vi "Oven_Con_Status.vi"() -> ()   [LabVIEW 2017]
uses:
  99af3ae5-4f0b-4404-ba7d-ed1d743938f4.vi
  <vilib>/addons/database/Connection.llb/DB Tools Open Connec (Path).vi
  <vilib>/addons/database/NI_Database_API.lvlib
panel:
  out "subarray":string[](array[string])
  out "index of element":i32
  out "output array":string[](array[string])
  out "data":string[][](array[string])
  out "error out 4":errorcluster
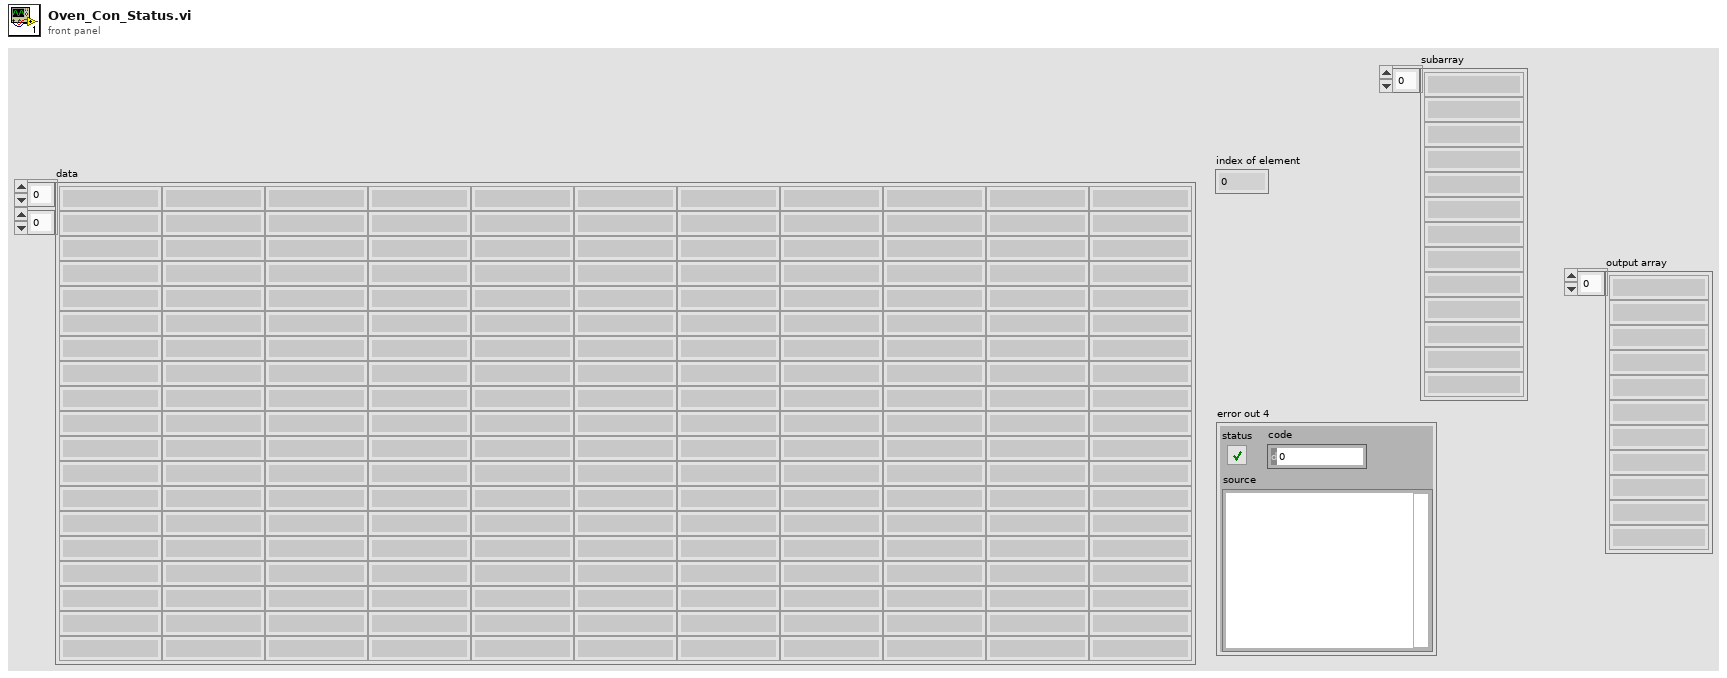
[diagram p1: front panel]
types:
  T1 = typedef "NI_Database_API.lvlib/Conn ObjectReference.ctl" = refnum<k1>
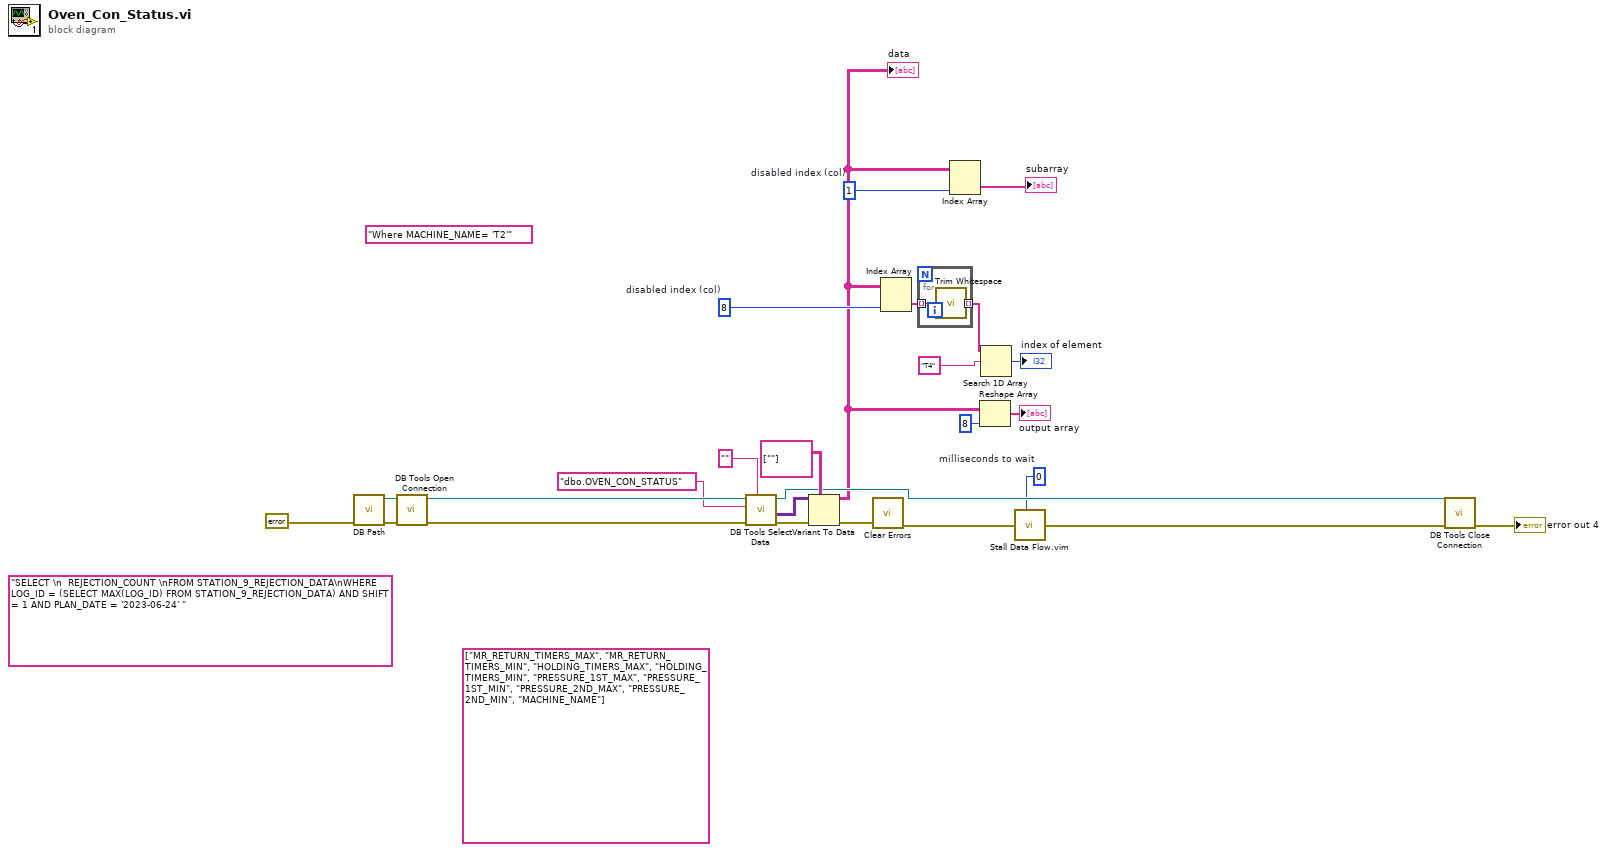
[diagram p0: block diagram]
diagram:
  w2 = 1  # disabled index (col)
  w9 = 8  # disabled index (col)
  w13 = u32 0  # milliseconds to wait
  (unwired) string[] ["MR_RETURN_TIMERS_MAX", "MR_RETURN_TIMERS_MIN", "HOLDING_TIMERS_MAX", "HOLDING_TIMERS_MIN", "PRESSURE_1ST_MAX", "PRESSURE_1ST_MIN", "PRESSURE_2ND_MAX", "PRESSURE_2ND_MIN", "MACHINE_NAME"] ("String")
  (unwired) "Where MACHINE_NAME= 'T2'" ("condition")
  (unwired) "SELECT \n  REJECTION_COUNT \nFROM STATION_9_REJECTION_DATA\nWHERE LOG_ID = (SELECT MAX(LOG_ID) FROM STATION_9_REJECTION_DATA) AND SHIFT = 1 AND PLAN_DATE = '2023-06-24' " ("SQL query")
  n1 = call "DB Path.vi"("error in"=errorcluster {"status"=FALSE, "code"=0, "source"=""} ("error in (no error)")) -> ("error out"=w21:errorcluster, "DB Path"=w22:path)  [unwired: 9 in]
  n2 = call-poly <vilib>:"DB Tools Open Connection.vi"("error in (no error)"=w21, "connection information"=w22) -> ("error out"=w16:errorcluster, "connection reference"=w20:T1)  [unwired: 6 in]
  n3 = call <vilib>:"DB Tools Select Data.vi"("condition"="", "error in (no error)"=w16, "table"="dbo.OVEN_CON_STATUS", "connection reference"=w20) -> ("error out"=w26:errorcluster, "data"=w25:variant[][], "connection reference out"=w18:T1)  [unwired: 2 in]
  n4 = Variant To Data(error in=w26, type=string[][] [[""]], Variant=w25) -> (data=w3:string[][], error out=w23:errorcluster)
  "data" <- w3
  n5 = call <vilib>:"Clear Errors.vi"("error in (no error)"=w23) -> ("error out"=w15:errorcluster)  [unwired: 5 in, 1 out]
  n6 = Index Array(array=w3, index (col)=w9) -> (element=w8:string[])  [unwired: 1 in]
  n7 = for {
    tunnel: w8 -> [w28] mode=indexing
    tunnel: [w27] -> w4 mode=indexing
    n8 = call <vilib>:"Trim Whitespace.vi"("string"=w28) -> ("trimmed string"=w27:string)  [unwired: 1 in]
  }
  n9 = Index Array(array=w3, index (col)=w2) -> (element=→"subarray":string[])  [unwired: 1 in]
  n10 = Reshape Array(w3, 8 ("dimension size")) -> (→"output array":string[])
  n11 = Search 1D Array(1D array=w4, element="T4" ("condition")) -> (index of element=→"index of element":i32)  [unwired: 1 in]
  n12 = call "Stall Data Flow.vim"("value in"=w15, "milliseconds to wait"=w13) -> ("value out"=w14:errorcluster)  [unwired: 1 out]
  n13 = call <vilib>:"DB Tools Close Connection.vi"("error in (no error)"=w14, "connection reference"=w18) -> ("error out"=→"error out 4":errorcluster)  [unwired: 5 in]
